vi "Track2.vi"() -> ()   [LabVIEW 2011]
doc: "This VI demonstrates how to control the Robotics Starter Kit 1.0 robot. It is deployed to an sbRIO-9631, then run on the Real-Time controller."
uses:
  <vilib>/Platform/TimedLoop/XDataNode/timing_clust.ctl
  <vilib>/Platform/TimedLoop/XDataNode/nitl_modes.ctl
  <vilib>/Platform/TimedLoop/XDataNode/wakeup.ctl
  <vilib>/robotics/Starter Kit/1.0/9631 Host Interface/NI_Robotics_Starter Kit Host_9631_1.0.lvclass
  <vilib>/Analysis/Matrix/Numeric/Conversions/Array To Matrix - RA.vi
  <vilib>/Platform/TimedLoop/XDataNode/XDataNode.xnode
  <vilib>/Platform/TimedLoop/XDataNode/XDNodeRunTimeDep.lvlib
  <vilib>/Analysis/Matrix/NI_Matrix.lvlib
  <vilib>/robotics/Starter Kit/Host Interface/NI_Robotics_Starter Kit Host.lvclass
panel:
  out "Vr/Wr":dbl[](array[numeric])
  out "Phi":dbl[](array[numeric])
  out "Iteracion":i32
  out "Vl/Q":dbl[](array[numeric])
  out "Boolean":bool
  out "PhiL":dbl
  out "PhiR":dbl
  out "X-Y 4":cluster{dbl[], dbl[]}(graph)
  out "W":cluster{dbl[], dbl[]}(graph)
  out "VL":cluster{dbl[], dbl[]}(graph)
  in  "Kp W":dbl step=0.01
  in  "Kp VL":dbl step=0.01
  in  "Paso":dbl
  in  "Tiempo":dbl
  in  "stop":bool
  out "X-Y":cluster{dbl[], dbl[]}(graph)
  out "Xr - X":dbl[](array[numeric])
  out "Zigma":dbl[](array[numeric])
  out "Zigmar":dbl[](array[numeric])
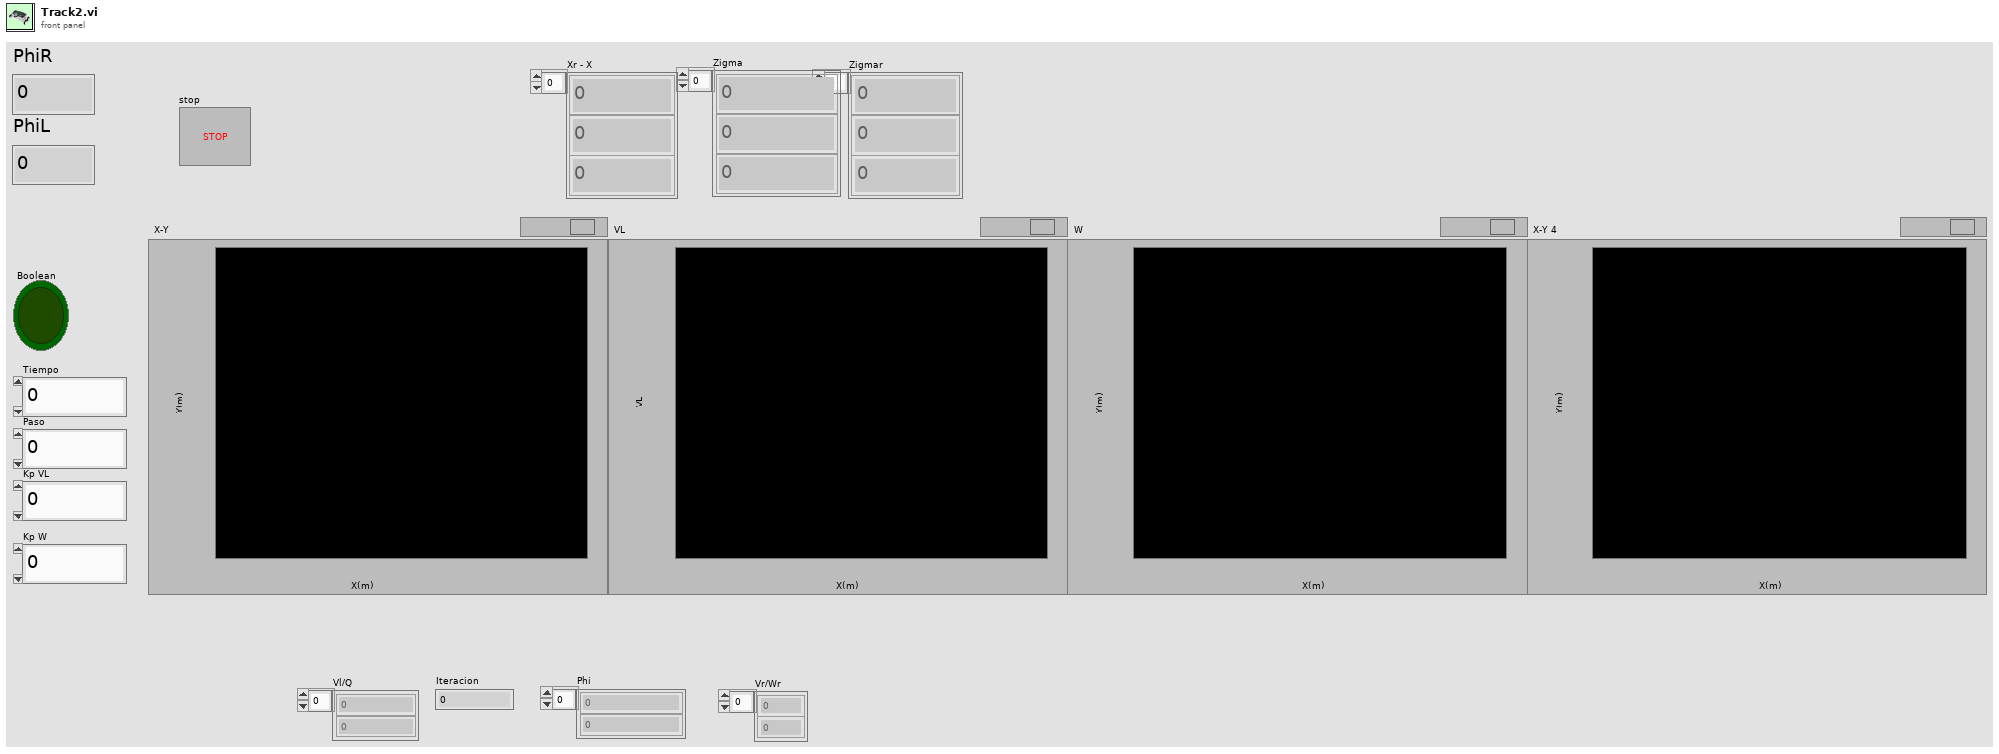
[diagram p1: front panel]
types:
  T1 = typedef "NI_Matrix.lvlib/RealMatrix.ctl" = dbl[][]
  T2 = typedef "XDNodeRunTimeDep.lvlib/timing_clust.ctl" = cluster{"Expected End [f-1]":u64, "Actual End [f-1]":u64, "Finished Late? [f-1]":bool, "Expected End [i-1]":u64, "Actual End [i-1]":u64, "Finished Late? [i-1]":bool, "Expected Start [i]":u64, "Actual Start [i]":u64, "Expected Start [f]":u64, "Actual Start [f]":u64, "Source Name":string, "Structure Name":string, "Period":i64, "Deadline":i64, "Offset":i64, "Start":i64, "Priority":i32, "Timeout":i32, "Mode":T3, "Wakeup Reason":T4, "Error":errorcluster, "Source Type":string, "Secondary Source Type":string, "Global End Time":u64, "Global Start Time":u64, "Frame Duration":u64, "Iteration Duration":u64, "Assigned CPU":i32, "I/O Scan Engine Mode":u32}
  T3 = typedef "XDNodeRunTimeDep.lvlib/nitl_modes.ctl" = enum32{"No Change", "Process missed periods, maintain original phase", "Discard missed periods, maintain original phase", "Process missed periods, ignore original phase", "Discard missed periods, ignore original phase"}
  T4 = typedef "XDNodeRunTimeDep.lvlib/wakeup.ctl" = enum32{"Normal", "Aborted", "Asynchronous wakeup", "Timing source error", "Timed loop error", "Timeout"}
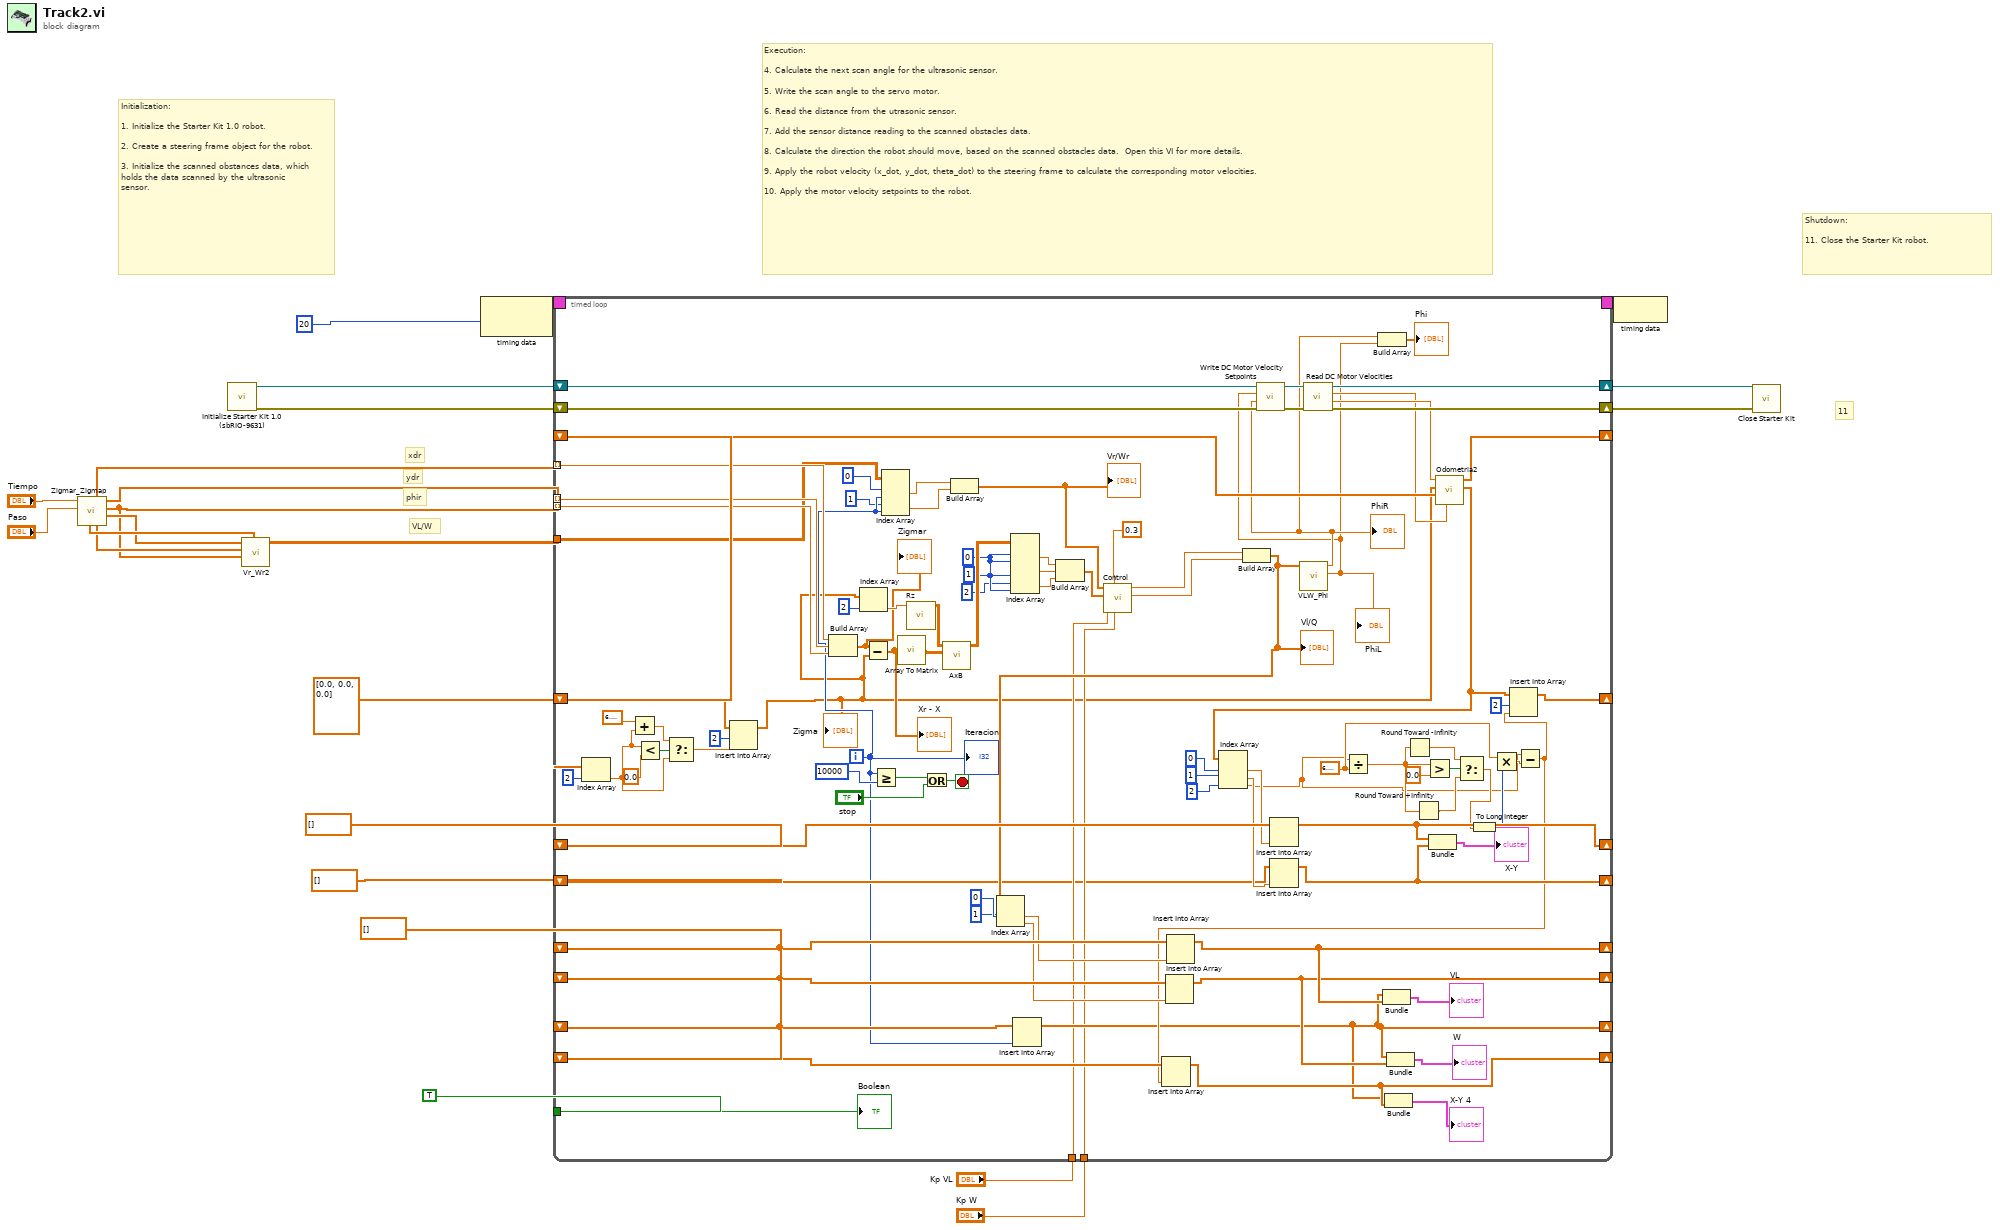
[diagram p0: block diagram]
diagram:
  w9 = dbl[] []
  w16 = dbl[] [0.0, 0.0, 0.0]
  # "VL/W"
  # "phir"
  # "ydr"
  # "xdr"
  # "11"
  # "Shutdown:\n\n11. Close the Starter Kit robot."
  # "Execution:\n\n4. Calculate the next scan angle for the ultrasonic sensor.\n\n5. Write the scan angle to the servo motor.\n\n6. Read the distance from the utrasonic sensor.\n\n7. Add the sensor distance reading to the scanned obstacles data.\n\n8. Calculate the direction the robot should move, based on the scanned obstacles data.  Open this VI for more details.\n\n9. Apply the robot velocity (x_dot, y_dot, theta_dot) to the steering frame to calculate the corresponding motor velocities.\n\n10. Apply the motor velocity setpoints to the robot."
  # "Initialization:\n\n1. Initialize the Starter Kit 1.0 robot.\n\n2. Create a steering frame object for the robot.\n\n3. Initialize the scanned obstances data, which holds the data scanned by the ultrasonic sensor."
  n1 = call "Zigmar_Zigmap.vi"("Paso"="Paso", "Tiempo"="Tiempo") -> ("Xdrp"=w3:dbl[], "Phir"=w1:dbl[], "Ydr"=w8:dbl[], "Ydrp"=w2:dbl[], "Xdr"=w7:dbl[], "Phirp"=w4:dbl[])  [unwired: 4 in]
  n2 = call <vilib>:"Initialize Starter Kit 1.0 (sbRIO-9631).vi"() -> ("error out"=w13:errorcluster, "FPGA starter kit host 1.0 out"=w12:refnum<class "NI_Robotics_Starter Kit Host_9631_1.0.lvclass">)  [unwired: 10 in]
  n3 = call "Vr_Wr2.vi"("Phirp"=w4, "Phir"=w1, "Ydrp"=w2, "Xdrp"=w3) -> ("VLW"=w5:T1)  [unwired: 7 in]
  n4 = node-c288(i64 20 ("Period")) -> (w23:T2)
  n5 = timed-loop {
    shift-right: [w106] -> w10
    shift-left: w12 -> [w108]
    shift-right: [w105] -> w11
    shift-left: w13 -> [w107]
    timing: w23 -> [_]
    timing-out: [_] -> w22
    tunnel: w7 -> [w120] mode=indexing
    tunnel: w8 -> [w119] mode=indexing
    tunnel: w1 -> [w118] mode=indexing
    shift-right: [w88] -> _
    shift-left: w16 -> [w25]
    tunnel: "Kp VL" -> [w50]
    tunnel: "Kp W" -> [w49]
    shift-right: [w101] -> _
    shift-left: w16 -> [w102]
    shift-right: [w95] -> _
    shift-left: dbl[] [] -> [w100]
    shift-right: [w94] -> _
    shift-left: dbl[] [] -> [w46]
    shift-right: [w67] -> _
    shift-left: w9 -> [w76]
    shift-right: [w64] -> _
    shift-left: w9 -> [w71]
    shift-right: [w61] -> _
    shift-left: w9 -> [w66]
    shift-right: [w63] -> _
    shift-left: w9 -> [w65]
    tunnel: w5 -> [w42]
    tunnel: TRUE -> [w38]
    i -> [w45]
    stop <- w115 stop-if-true
    w57 = 0 ("index (col)")
    w87 = 6.283185307179586
    n6 = Index Array(array=w25, index=2) -> (element=w28:dbl)
    n7 = Add(x=6.283185307179586, y=w28) -> (x+y=w30:dbl)
    n8 = Less?(x=w28, y=0.0) -> (x < y?=w33:bool)
    n9 = Select(t=w30, s=w33, f=w28) -> (s? t:f=w27:dbl)
    n10 = Insert Into Array(array=w25, index=2, new element=w27) -> (w24:dbl[])
    "Zigma" <- w24
    n11 = Build Array(w120, w119, w118) -> (w34:dbl[])
    "Zigmar" <- w34
    n12 = Index Array(array=w24, index=2) -> (element=w117:dbl)
    n13 = Subtract(x=w34, y=w24) -> (x-y=w112:dbl[])
    "Xr - X" <- w112
    n14 = Greater Or Equal?(x=w45, y=10000 ("x")) -> (x >= y?=w103:bool)
    n15 = Index Array(array=w42, index (row) #1=0 ("index (row)"), index (col) #1=w45, index (row) #2=1 ("index (row)"), index (col) #2=w45) -> (element #1=w41:dbl, element #2=w40:dbl)
    n16 = call-poly <vilib>:"Array To Matrix.vi"("Real 1D Array"=w112) -> ("Real Matrix (Column Vector)"=w111:T1)
    n17 = call "Rz.vi"("theta"=w117) -> ("RotacionalZ"=w113:T1)  [unwired: 10 in]
    n18 = Or(x=w103, y="stop") -> (x .or. y?=w115:bool)
    n19 = call "AxB.vi"("B"=w111, "A"=w113) -> ("AxB"=w58:T1)  [unwired: 9 in]
    n20 = Build Array(w41, w40) -> (w39:dbl[])
    "Vr/Wr" <- w39
    n21 = Index Array(array=w58, index (row) #1=w57, index (col) #1=w57, index (row) #2=1 ("index (row)"), index (col) #2=w57, index (row) #3=2 ("index (row)"), index (col) #3=w57) -> (element #1=w54:dbl, element #2=w53:dbl, element #3=w52:dbl)
    n22 = Insert Into Array(array=w66, new element=w45) -> (w61:dbl[])  [unwired: 1 in]
    n23 = Build Array(w54, w53, w52) -> (w51:dbl[])
    n24 = call "Control.vi"("Kp2"=w49, "Q"=0.3, "KV"=w50, "Zigmae"=w51, "Vr/Wr"=w39) -> ("W"=w47:dbl, "V"=w48:dbl)  [unwired: 5 in]
    n25 = Build Array(w48, w47) -> (w75:dbl[])
    "Vl/Q" <- w75
    n26 = Index Array(array=w75, index #1=0 ("index"), index #2=1 ("index")) -> (element #1=w72:dbl, element #2=w70:dbl)
    n27 = Insert Into Array(array=w71, new element=w70) -> (w64:dbl[])  [unwired: 1 in]
    n28 = Insert Into Array(array=w76, new element=w72) -> (w67:dbl[])  [unwired: 1 in]
    n29 = call "VLW_Phi.vi"("VL/W"=w75) -> ("PhiL"=w36:dbl, "PhiR"=w37:dbl)  [unwired: 9 in]
    "PhiR" <- w37
    "PhiL" <- w36
    n30 = call <vilib>:"Write DC Motor Velocity Setpoints.vi"("error in (no error)"=w107, "right motor ccw velocity (rad/s)"=w37, "left motor ccw velocity (rad/s)"=w36, "starter kit host in"=w108) -> ("error out"=w110:errorcluster, "starter kit host out"=w109:refnum<class "NI_Robotics_Starter Kit Host_9631_1.0.lvclass">)  [unwired: 6 in]
    n31 = call <vilib>:"Read DC Motor Velocities.vi"("error in (no error)"=w110, "starter kit host in"=w109) -> ("error out"=w105:errorcluster, "right motor ccw velocity (rad/s)"=w92:dbl, "left motor ccw velocity (rad/s)"=w91:dbl, "starter kit host out"=w106:refnum<class "NI_Robotics_Starter Kit Host_9631_1.0.lvclass">)  [unwired: 6 in]
    n32 = Build Array(w37, w36) -> (→"Phi":dbl[])
    n33 = Bundle(w61, w67) -> (→"VL":cluster{dbl[], dbl[]})  [unwired: 1 in]
    n34 = Bundle(w61, w64) -> (→"W":cluster{dbl[], dbl[]})  [unwired: 1 in]
    n35 = call "Odometria2.vi"("left motor ccw velocity (rad/s)"=w91, "Arrastrado"=w102, "Zigma"=w24, "right motor ccw velocity (rad/s)"=w92) -> ("Array out"=w89:dbl[], "Arrastrad_out"=w101:dbl[])  [unwired: 6 in]
    n36 = Index Array(array=w89, index #1=0 ("index"), index #2=1 ("index"), index #3=2 ("index")) -> (element #1=w97:dbl, element #2=w96:dbl, element #3=w78:dbl)
    n37 = Insert Into Array(array=w100, new element=w97) -> (w95:dbl[])  [unwired: 1 in]
    n38 = Insert Into Array(array=w46, new element=w96) -> (w94:dbl[])  [unwired: 1 in]
    n39 = Divide(x=w78, y=w87) -> (x/y=w82:dbl)
    n40 = Round Toward -Infinity(1:w82) -> (0:w84:dbl)
    n41 = Round Toward +Infinity(x=w82) -> (ceil(x): smallest int >= x=w81:dbl)
    n42 = Greater?(x=w82, y=0.0) -> (0:w86:bool)
    n43 = Bundle(w95, w94) -> (→"X-Y":cluster{dbl[], dbl[]})  [unwired: 1 in]
    n44 = Select(t=w84, s=w86, f=w81) -> (s? t:f=w79:dbl)
    n45 = To Long Integer(number=w79) -> (32bit integer=w80:i32)
    n46 = Multiply(x=w87, y=w80) -> (x*y=w85:dbl)
    n47 = Subtract(x=w78, y=w85) -> (x-y=w62:dbl)
    n48 = Insert Into Array(array=w65, new element=w62) -> (w63:dbl[])  [unwired: 1 in]
    n49 = Bundle(w61, w63) -> (→"X-Y 4":cluster{dbl[], dbl[]})  [unwired: 1 in]
    n50 = Insert Into Array(array=w89, index=2, new element=w62) -> (w88:dbl[])
    "Boolean" <- w38
    "Iteracion" <- w45
  }
  n51 = node-c288(w22) -> ()
  n52 = call-dynamic "Close Starter Kit.vi"("error in (no error)"=w11, "starter kit host in"=w10) -> ()  [unwired: 9 in, 1 out]
